vi "Configure Arming (Auto).vi"(0 "VISA resource name":refnum<visa-resource-name>, 1 "Measurement (0:Frequency)":i32(ring) items=["Frequency", "Frequency Ratio", "Period", "Totalize", "Phase", "Edge Rise Time", "Edge Fall Time", "Positive Pulse Width", "Negative Pulse Width", "Duty Cycle", "Time Interval", "Volt Maximum", "Volt Minimum"], 11 "error in (no error)":errorcluster, 12 "Time Interval":cluster{"Delay Type":i32, "Delay Value (0)":dbl} {"Delay Type" items=["None", "Time", "Event"]}) -> (4 "VISA resource name out":refnum<visa-resource-name>, 15 "error out":errorcluster)   [LabVIEW 2020, in "Counter.lvlib" / "PICOTEST U62XXA series.lvlib"]
doc: "Configures Auto Arming Settings. This VI should be called after the Configure Measurement VI.\n\n<B>Note:</B>\n\nVolt Peak Measurements <B>does not</B> have Auto Arming capabilities."
uses:
  PICOTEST U62XXA series.lvlib
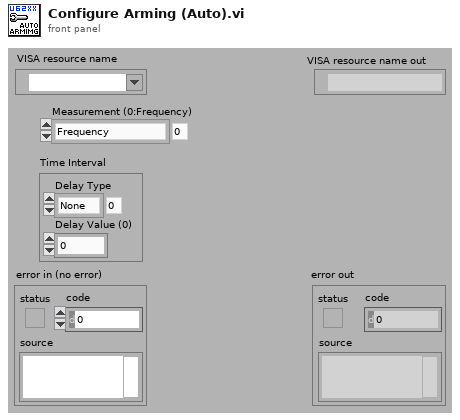
[diagram p1: front panel]
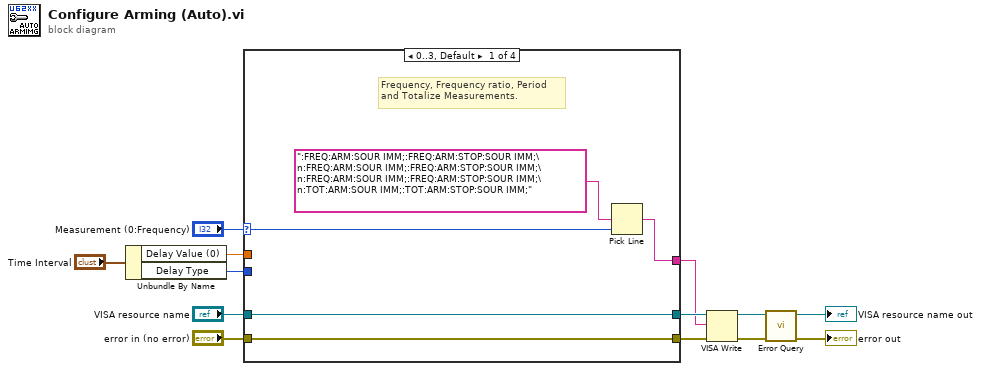
[diagram p0: block diagram]
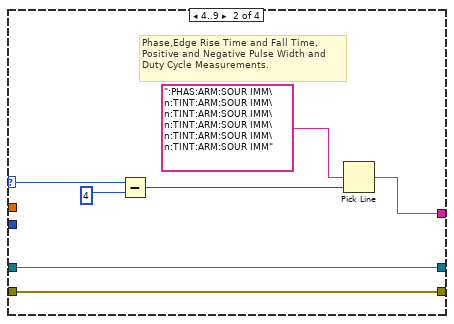
[diagram p2: hidden frame]
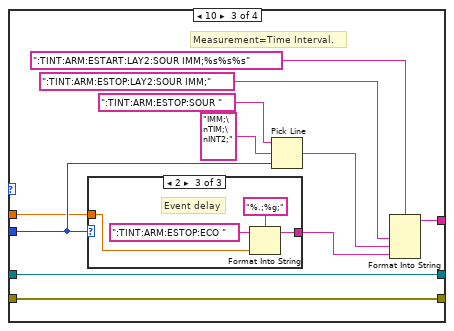
[diagram p3: hidden frame]
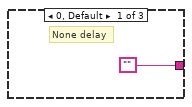
[diagram p4: hidden frame]
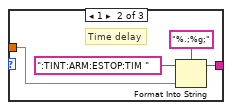
[diagram p5: hidden frame]
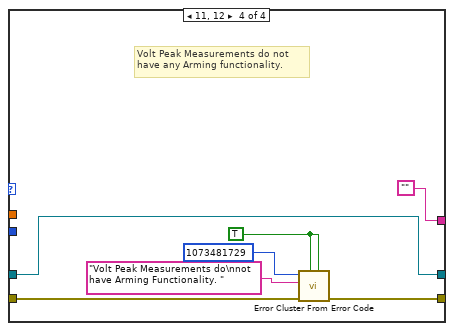
[diagram p6: hidden frame]
diagram:
  n1 = Unbundle By Name("Time Interval") -> ("Delay Value (0)"=w7:dbl, "Delay Type"=w6:i32)
  n2 = case shown="0..3, Default" "Measurement (0:Frequency)" {
    selector: "Measurement (0:Frequency)" -> [w18 w23 _ _]
    tunnel: [w14 w19 w30 ""] -> w1
    tunnel: w7 -> [_ _ w33 _]
    tunnel: w6 -> [_ _ w34 _]
    tunnel: [w17 w21 w32 w49] -> w4
    tunnel: "VISA resource name" -> [w17 w21 w32 w49]
    tunnel: "error in (no error)" -> [w16 w20 w31 w48]
    tunnel: [w16 w20 w31 w50] -> w2
    frame 0..3, Default {
      # "Frequency, Frequency ratio, Period\nand Totalize Measurements."
      n3 = Pick Line(multi-line string=":FREQ:ARM:SOUR IMM;:FREQ:ARM:STOP:SOUR IMM;\n:FREQ:ARM:SOUR IMM;:FREQ:ARM:STOP:SOUR IMM;\n:FREQ:ARM:SOUR IMM;:FREQ:ARM:STOP:SOUR IMM;\n:TOT:ARM:SOUR IMM;:TOT:ARM:STOP:SOUR IMM;" ("string (\"\")"), line index=w18) -> (output string=w14:string)  [unwired: 1 in]
    }
    frame 4..9 {
      # "Phase,Edge Rise Time and Fall Time,\nPositive and Negative Pulse Width and\nDuty Cycle Measurements."
      n4 = Subtract(x=w23, y=4) -> (x-y=w22:i32)
      n5 = Pick Line(multi-line string=":PHAS:ARM:SOUR IMM\n:TINT:ARM:SOUR IMM\n:TINT:ARM:SOUR IMM\n:TINT:ARM:SOUR IMM\n:TINT:ARM:SOUR IMM\n:TINT:ARM:SOUR IMM", line index=w22) -> (output string=w19:string)  [unwired: 1 in]
    }
    frame 10 {
      # "Measurement=Time Interval."
      n6 = case shown="2" w34 {
        tunnel: w33 -> [_ w39 w42]
        tunnel: ["" w38 w44] -> w26
        frame 0, Default {
          # "None delay"
        }
        frame 1 {
          # "Time delay"
          n7 = Format Into String(format string="%.;%g;", initial string=":TINT:ARM:ESTOP:TIM ", w39) -> (resulting string=w38:string)  [unwired: 1 in, 1 out]
        }
        frame 2 {
          # "Event delay"
          n8 = Format Into String(format string="%.;%g;", initial string=":TINT:ARM:ESTOP:ECO ", w42) -> (resulting string=w44:string)  [unwired: 1 in, 1 out]
        }
      }
      n9 = Pick Line(string ("")=":TINT:ARM:ESTOP:SOUR ", multi-line string="IMM;\nTIM;\nINT2;", line index=w34) -> (output string=w27:string)
      n10 = Format Into String(format string=":TINT:ARM:ESTART:LAY2:SOUR IMM;%s%s%s", ":TINT:ARM:ESTOP:LAY2:SOUR IMM;", w27, w26) -> (resulting string=w30:string)  [unwired: 2 in, 1 out]
    }
    frame 11, 12 {
      w52 = TRUE ("is warning? (False)")
      # "Volt Peak Measurements do not \nhave any Arming functionality."
      n11 = call <vilib>:"Error Cluster From Error Code.vi"("is warning? (False)"=w52, "show call chain? (False)"=w52, "error in (no error)"=w48, "error message (\"\")"="Volt Peak Measurements do\nnot have Arming Functionality. " ("error message (\"\")"), "error code (0)"=1073481729 ("Code")) -> ("error out"=w50:errorcluster)  [unwired: 4 in]
    }
  }
  n12 = VISA Write(VISA resource name=w4, write buffer=w1, error in (no error)=w2) -> (VISA resource name out=w12:refnum<visa-resource-name>, error out=w11:errorcluster)  [unwired: 1 out]
  n13 = call "Error Query.vi"("error in (no error)"=w11, "VISA resource name"=w12) -> ("error out"=→"error out":errorcluster, "VISA resource name out"=→"VISA resource name out":refnum<visa-resource-name>)  [unwired: 6 in, 2 out]
